vi "Home Correction.vi"() -> (0 "RL Dist":dbl, 1 "Angle out":dbl, 3 "Close Range":dbl)   [LabVIEW 2018]
panel:
  out "X1":dbl
  out "X2":dbl
  out "Y2":dbl
  out "Y1":dbl
  out "Block rad":dbl
  out "Index Counter A":i32
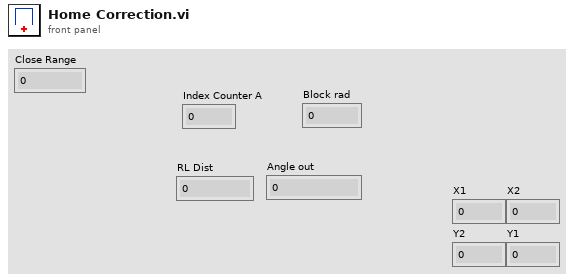
[diagram p1: front panel]
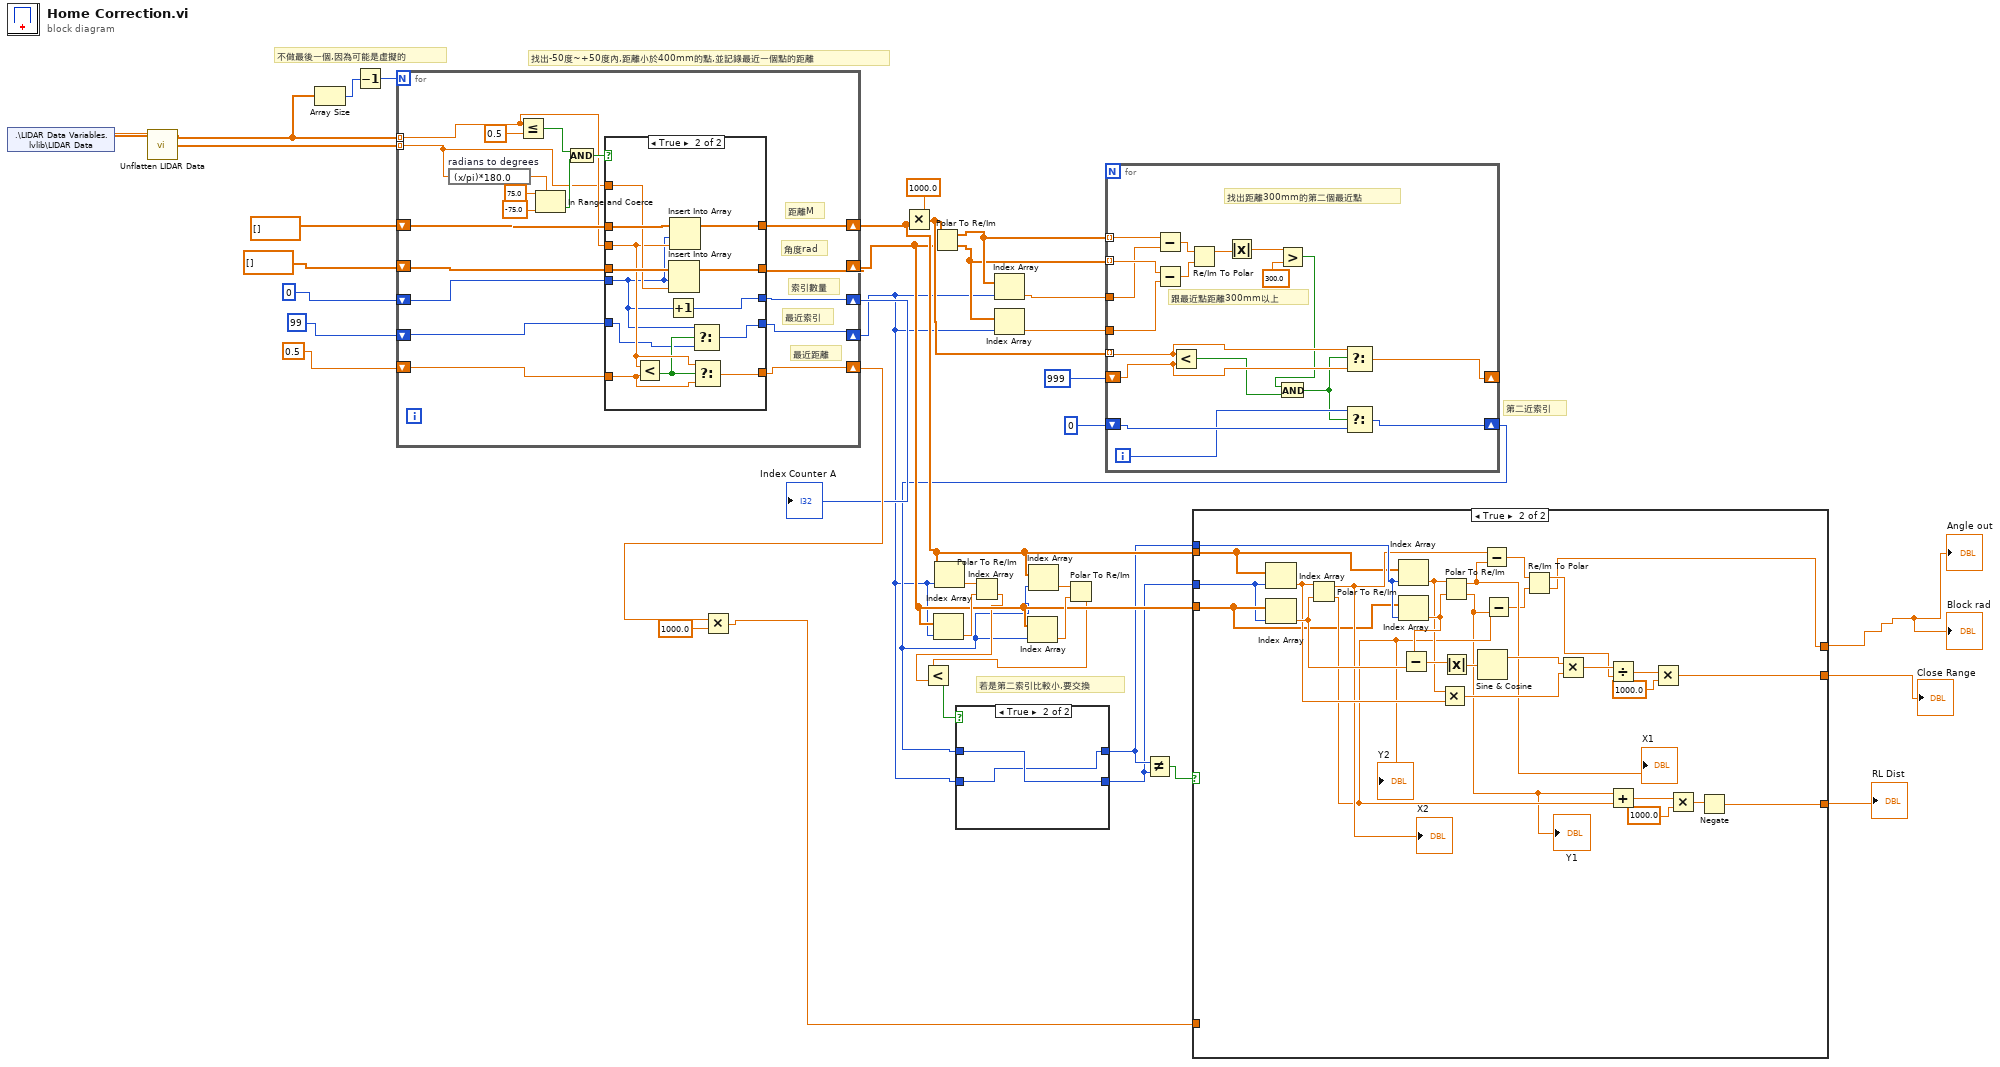
[diagram p0: block diagram]
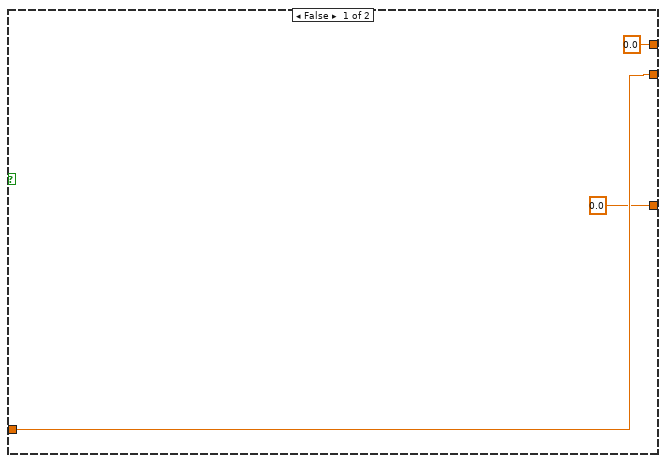
[diagram p3: hidden frame]
diagram:
  # "不做最後一個,因為可能是虛擬的"
  # "若是第二索引比較小,要交換"
  # "第二近索引"
  # "找出-50度~+50度內,距離小於400mm的點,並記錄最近一個點的距離"
  n1 = shared-variable ".\\LIDAR Data Variables.lvlib\\LIDAR Data"() -> (w34:dbl[])  [unwired: 1 in, 1 out]
  n2 = call "Unflatten LIDAR Data.vi"("Flat LIDAR Data"=w34) -> ("Bearing (rad)"=w33:dbl[], "Range (m)"=w17:dbl[])  [unwired: 7 in, 2 out]
  n3 = Array Size(array=w17) -> (size(s)=w15:i32)
  n4 = Decrement(x=w15) -> (x-1=w16:i32)
  n5 = for {
    N: w16 -> [_]
    tunnel: w17 -> [w42] mode=indexing
    tunnel: w33 -> [w41] mode=indexing
    shift-right: [w49] -> w10
    shift-left: dbl[] [] -> [w52]
    shift-right: [w48] -> w9
    shift-left: dbl[] [] -> [w51]
    shift-right: [w43] -> w29
    shift-left: 0 -> [w50]
    shift-right: [w45] -> w31
    shift-left: 0.5 -> [w47]
    shift-right: [w44] -> w5
    shift-left: 99 -> [w46]
    # "索引數量"
    # "最近距離"
    # "最近索引"
    # "角度rad"
    # "距離M"
    n6 = expression code="(x/pi)*180.0" "radians to degrees"(w41) -> (w40:dbl)
    n7 = Less Or Equal?(x=w42, y=0.5) -> (x <= y?=w55:bool)
    n8 = In Range and Coerce(upper limit=75.0, x=w40, lower limit=-75.0) -> (In Range?=w54:bool)  [unwired: 1 out]
    n9 = And(x=w55, y=w54) -> (x .and. y?=w53:bool)
    n10 = case shown="True" w53 {
      tunnel: w52 -> [w63 w76]
      tunnel: w51 -> [w62 w75]
      tunnel: w50 -> [w59 w65]
      tunnel: w42 -> [_ w70]
      tunnel: w41 -> [_ w74]
      tunnel: [w63 w73] -> w49
      tunnel: [w62 w72] -> w48
      tunnel: w47 -> [w61 w71]
      tunnel: w46 -> [w60 w67]
      tunnel: [w61 w69] -> w45
      tunnel: [w60 w66] -> w44
      tunnel: [w59 w64] -> w43
      frame False {
      }
      frame True {
        n11 = Less?(x=w70, y=w71) -> (x < y?=w68:bool)
        n12 = Increment(x=w65) -> (x+1=w64:i32)
        n13 = Insert Into Array(array=w75, index=w65, new element=w74) -> (w72:dbl[])
        n14 = Insert Into Array(array=w76, index=w65, new element=w70) -> (w73:dbl[])
        n15 = Select(t=w65, s=w68, f=w67) -> (s? t:f=w66:i32)
        n16 = Select(t=w70, s=w68, f=w71) -> (s? t:f=w69:dbl)
      }
    }
  }
  "Index Counter A" <- w29
  n17 = Multiply(x=w31, y=1000.0) -> (x*y=w20:dbl)
  n18 = Multiply(x=1000.0 ("upper limit"), y=w10) -> (x*y=w24:dbl[])
  n19 = Polar To Re/Im(2:w9, 3:w24) -> (0:w22:dbl[], 1:w23:dbl[])
  n20 = Index Array(array=w9, index=w5) -> (element=w13:dbl)
  n21 = Index Array(array=w10, index=w5) -> (element=w14:dbl)
  n22 = Polar To Re/Im(2:w13, 3:w14) -> (0:w7:dbl)  [unwired: 1 out]
  n23 = Index Array(array=w23, index=w5) -> (element=w27:dbl)
  n24 = Index Array(array=w22, index=w5) -> (element=w28:dbl)
  n25 = for {
    tunnel: w23 -> [w94] mode=indexing
    tunnel: w22 -> [w93] mode=indexing
    tunnel: w28 -> [w92]
    tunnel: w27 -> [w91]
    tunnel: w24 -> [w87] mode=indexing
    shift-right: [w85] -> _
    shift-left: 999 -> [w86]
    shift-right: [w82] -> w6
    shift-left: 0 -> [w84]
    i -> [w83]
    # "找出距離300mm的第二個最近點"
    # "跟最近點距離300mm以上"
    n26 = Subtract(x=w94, y=w91) -> (x-y=w90:dbl)
    n27 = Subtract(x=w93, y=w92) -> (x-y=w89:dbl)
    n28 = Less?(x=w87, y=w86) -> (x < y?=w80:bool)
    n29 = Re/Im To Polar(2:w89, 3:w90) -> (1:w78:dbl)  [unwired: 1 out]
    n30 = Absolute Value(x=w78) -> (abs(x)=w77:dbl)
    n31 = Greater?(x=w77, y=300.0) -> (0:w79:bool)
    n32 = And(x=w79, y=w80) -> (x .and. y?=w81:bool)
    n33 = Select(t=w87, s=w81, f=w86) -> (s? t:f=w85:dbl)
    n34 = Select(t=w83, s=w81, f=w84) -> (s? t:f=w82:i32)
  }
  n35 = Index Array(array=w9, index=w6) -> (element=w12:dbl)
  n36 = Index Array(array=w10, index=w6) -> (element=w11:dbl)
  n37 = Polar To Re/Im(2:w12, 3:w11) -> (0:w8:dbl)  [unwired: 1 out]
  n38 = Less?(x=w8, y=w7) -> (x < y?=w4:bool)
  n39 = case shown="True" w4 {
    tunnel: w6 -> [w96 w98]
    tunnel: w5 -> [w95 w97]
    tunnel: [w96 w97] -> w3
    tunnel: [w95 w98] -> w2
    frame False {
    }
    frame True {
    }
  }
  n40 = Not Equal?(x=w3, y=w2) -> (x != y?=w21:bool)
  n41 = case shown="True" w21 {
    tunnel: w3 -> [_ w129]
    tunnel: [w101 w116] -> w19
    tunnel: [0.0 w109] -> w18
    tunnel: w9 -> [_ w108]
    tunnel: w10 -> [_ w107]
    tunnel: w2 -> [_ w106]
    tunnel: w20 -> [w101 _]
    tunnel: [0.0 w102] -> w1
    frame False {
    }
    frame True {
      n42 = Index Array(array=w107, index=w106) -> (element=w123:dbl)
      n43 = Index Array(array=w108, index=w106) -> (element=w125:dbl)
      n44 = Polar To Re/Im(2:w125, 3:w123) -> (0:w111:dbl, 1:w112:dbl)
      "X2" <- w112
      "Y2" <- w111
      n45 = Index Array(array=w107, index=w129) -> (element=w124:dbl)
      n46 = Index Array(array=w108, index=w129) -> (element=w126:dbl)
      n47 = Subtract(x=w126, y=w125) -> (x-y=w127:dbl)
      n48 = Multiply(x=w124, y=w123) -> (x*y=w121:dbl)
      n49 = Polar To Re/Im(2:w126, 3:w124) -> (0:w103:dbl, 1:w115:dbl)
      "X1" <- w115
      "Y1" <- w103
      n50 = Absolute Value(x=w127) -> (abs(x)=w128:dbl)
      n51 = Sine & Cosine(0:w128) -> (1:w122:dbl)  [unwired: 1 out]
      n52 = Subtract(x=w112, y=w115) -> (x-y=w105:dbl)
      n53 = Subtract(x=w111, y=w103) -> (x-y=w104:dbl)
      n54 = Re/Im To Polar(2:w104, 3:w105) -> (0:w102:dbl, 1:w119:dbl)
      n55 = Multiply(x=w122, y=w121) -> (x*y=w120:dbl)
      n56 = Divide(x=w120, y=w119) -> (x/y=w118:dbl)
      n57 = Add(x=w103, y=w111) -> (x+y=w113:dbl)
      n58 = Multiply(x=w118, y=1000.0) -> (x*y=w116:dbl)
      n59 = Multiply(x=w113, y=1000.0) -> (x*y=w110:dbl)
      n60 = Negate(x=w110) -> (-x=w109:dbl)
    }
  }
  "Close Range" <- w19
  "RL Dist" <- w18
  "Angle out" <- w1
  "Block rad" <- w1
